vi "Get Scale Values.vi"(8 "error in (no error)":errorcluster, 11 "VISA resource name":refnum<visa-resource-name>) -> (0 "error out":errorcluster, 1 "Actual Full-scale Value":dbl format="%^.3e", 2 "Nominal Full-scale Value":dbl format="%^.3e", 3 "VISA resource name out":refnum<visa-resource-name>, 4 "Scale Units":i32)   [LabVIEW 2014, in "Fluke 5XXX Series Multicalibrators.lvlib"]
doc: "This VI returns the full-scale nominal and full-scale actual values set when SCALE more was turned on. If scaling is off, both responses one and two are \"0.0.\"\n\nNote:\n\nThis VI is available only for instrument models 5700A and 5720A."
uses:
  Fluke 5XXX Series Multicalibrators.lvlib
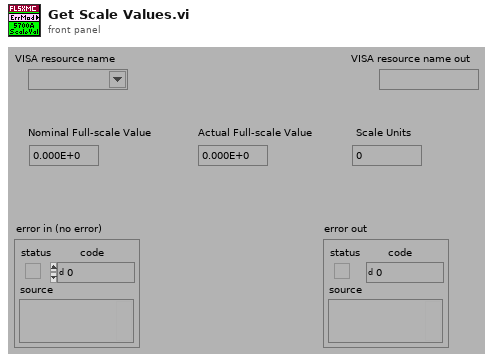
[diagram p1: front panel]
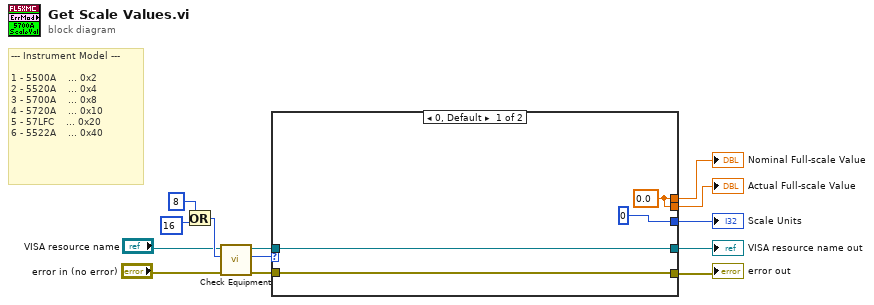
[diagram p0: block diagram]
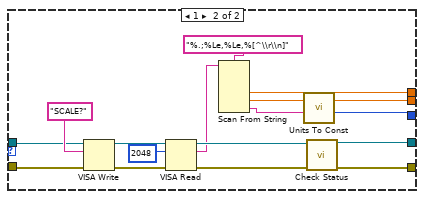
[diagram p2: hidden frame]
diagram:
  # "--- Instrument Model ---\n\n1 - 5500A    ... 0x2\n2 - 5520A    ... 0x4\n3 - 5700A    ... 0x8\n4 - 5720A    ... 0x10\n5 - 57LFC    ... 0x20\n6 - 5522A    ... 0x40"
  n1 = Or(x=8 ("Numeric"), y=16 ("Numeric")) -> (x .or. y?=w8:i32)
  n2 = call "Check Equipment.vi"("error in (no error)"="error in (no error)", "Bit Mask"=w8, "VISA resource name"="VISA resource name") -> ("error out"=w13:errorcluster, "Present?"=w12:u32, "VISA resource name out"=w11:refnum<visa-resource-name>)  [unwired: 6 in]
  n3 = case shown="0, Default" w12 {
    tunnel: [w17 w27] -> w5
    tunnel: [w16 w24] -> w4
    tunnel: w13 -> [w17 w29]
    tunnel: w11 -> [w16 w28]
    tunnel: [w14 w21] -> w1
    tunnel: [u16 0 w20] -> w3
    tunnel: [w14 w18] -> w2
    frame 0, Default {
      w14 = 0.0
    }
    frame 1 {
      n4 = VISA Write(VISA resource name=w28, write buffer="SCALE?", error in (no error)=w29) -> (VISA resource name out=w32:refnum<visa-resource-name>, error out=w31:errorcluster)  [unwired: 1 out]
      n5 = VISA Read(VISA resource name=w32, byte count=u32 2048 ("byte count (0)"), error in (no error)=w31) -> (VISA resource name out=w25:refnum<visa-resource-name>, read buffer=w22:string, error out=w26:errorcluster)  [unwired: 1 out]
      n6 = Scan From String(format string="%.;%Le,%Le,%[^\\r\\n]", input string=w22) -> (output 1=w21:dbl, output 2=w18:dbl, output 3=w19:string)  [unwired: 5 in, 3 out]
      n7 = call "Units To Const.vi"("Units"=w19) -> ("Const"=w20:i32)  [unwired: 10 in]
      n8 = call "Check Status.vi"("VISA resource name"=w25, "error in (no error)"=w26) -> ("VISA resource name out"=w24:refnum<visa-resource-name>, "error out"=w27:errorcluster)  [unwired: 12 in]
    }
  }
  "Nominal Full-scale Value" <- w1
  "Actual Full-scale Value" <- w2
  "Scale Units" <- w3
  "VISA resource name out" <- w4
  "error out" <- w5
